vi "acquisitionGetChannelsFromFrames.vi"(0 "frameIn":u16[][][](array[numeric])) -> (1 "Red":u16[][][](array[numeric]), 2 "Green":u16[][][](array[numeric]))   [LabVIEW 2017]
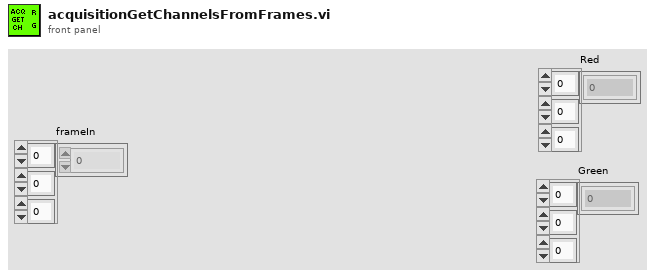
[diagram p1: front panel]
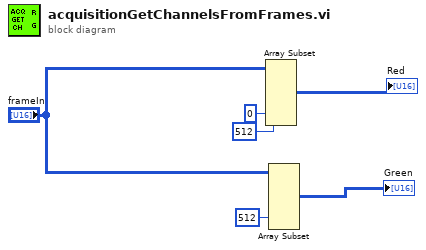
[diagram p0: block diagram]
diagram:
  n1 = Array Subset(array="frameIn", index (dim 2)=0 ("index"), length (dim 2)=512 ("length")) -> (→"Red":u16[][][])  [unwired: 4 in]
  n2 = Array Subset(array="frameIn", index (dim 2)=512 ("index")) -> (→"Green":u16[][][])  [unwired: 5 in]
